vi "Global_v20.vi"() -> ()   [LabVIEW 2021]
panel:
  out "VISA Powermeter":refnum<visa-resource-name> caption="instrument handle out"
  out "VISA Oceanoptics":refnum<visa-resource-name>
  # "Spectrometer"
  # "Power meter"
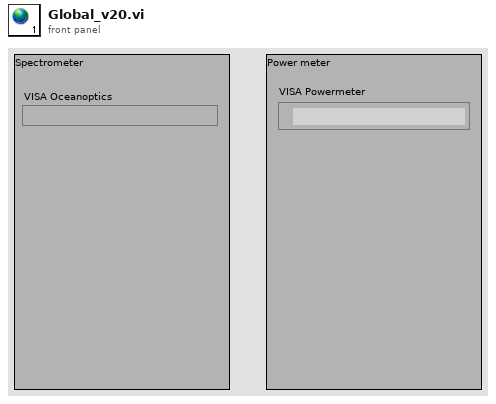
[diagram p1: front panel]
diagram:
